vi "test vi - Copy.vi"() -> ()   [LabVIEW 2018]
panel:
  out "Motor Error":errorcluster
  out "error out":errorcluster
  in  "stop":bool
  in  "wTargetSpeed":dbl
  in  "yTargetSpeed":dbl
  in  "xTargetSpeed":dbl
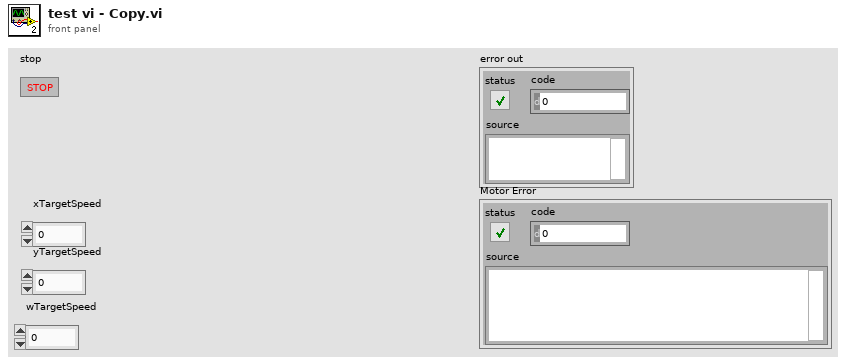
[diagram p1: front panel]
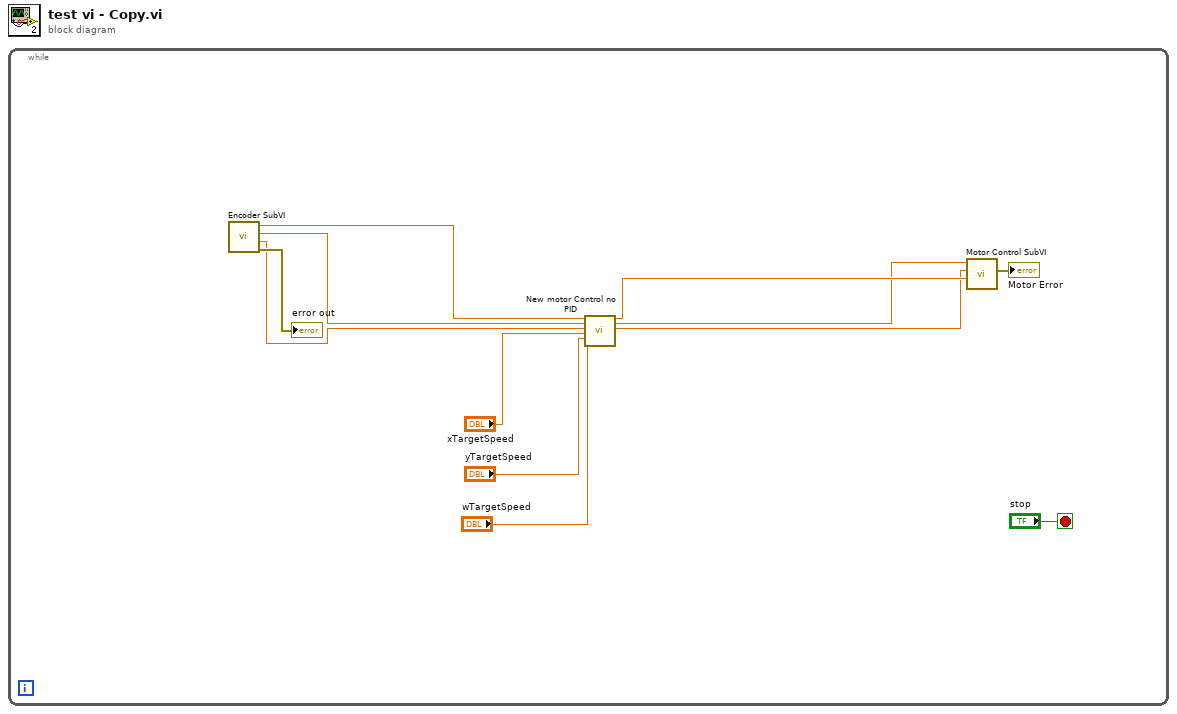
[diagram p0: block diagram]
diagram:
  n1 = while {
    stop <- "stop" stop-if-true
    n2 = call "Encoder SubVI.vi"() -> ("error out"=→"error out":errorcluster, "Distance M2"=w7:dbl, "Distance M1"=w8:dbl, "Distance M0"=w9:dbl)  [unwired: 8 in]
    n3 = call "New motor Control no PID.vi"("Encoder 0"=w9, "Encoder 1"=w8, "Encoder 2"=w7, "xTargetSpeed"="xTargetSpeed", "yTargetSpeed"="yTargetSpeed", "wTargetSpeed"="wTargetSpeed") -> ("M2"=w3:dbl, "M0"=w2:dbl, "M1"=w1:dbl)  [unwired: 11 in]
    n4 = call "Motor Control SubVI.vi"("Speed M2"=w3, "Speed M1"=w1, "Speed M0"=w2) -> ("Motor Error"=→"Motor Error":errorcluster)  [unwired: 8 in]
  }
